vi "comm transmit char.vi"(8 "error in (no error)":errorcluster, 10 "character to transmit":u8, 11 "Comm Handle":u64) -> (0 "error out":errorcluster, 3 "dup Comm Handle":u64)   [LabVIEW 2021, in "lvserial.lvlib"]
doc: "Transmits a specified character ahead of any pending data in the output buffer of the specified communications device."
uses:
  lvserial.lvlib
  lvserial.dll
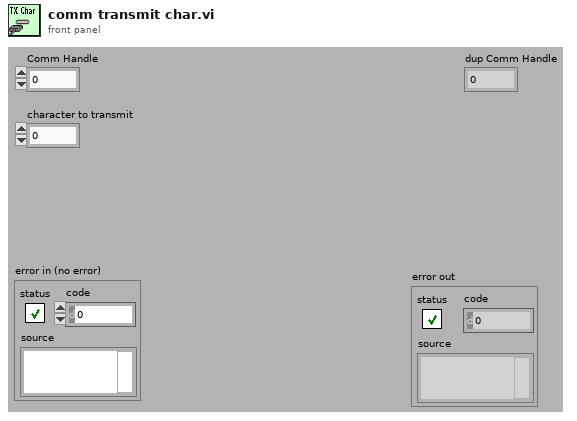
[diagram p1: front panel]
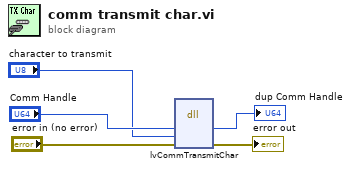
[diagram p0: block diagram]
diagram:
  n1 = dll-call lib="lvserial.dll" fn="lvCommTransmitChar"("hComm"="Comm Handle", "cChar"="character to transmit", "error"="error in (no error)") -> ("hComm"=→"dup Comm Handle":u64, "error"=→"error out":errorcluster)  [unwired: 4 in, 3 out]
